vi "DC.vi"(5 "结束冷却":bool, 6 "文本（TSDC）路径：":path=path "C:/Users/Scrooge/Desktop/TSDC.txt", 7 "Ctl Refnum":refnum<vi>, 8 "error in (no error)":errorcluster caption="错误输入（无错误）", 9 "结束温度":dbl, 10 "簇 2":T1, 11 "簇":T2) -> (0 "error out":errorcluster caption="错误输出", 2 "极化电流":dbl, 3 "簇 3":cluster{"当前温度":dbl, "当前电压":bool, "剩余时间":dbl})   [LabVIEW 2017]
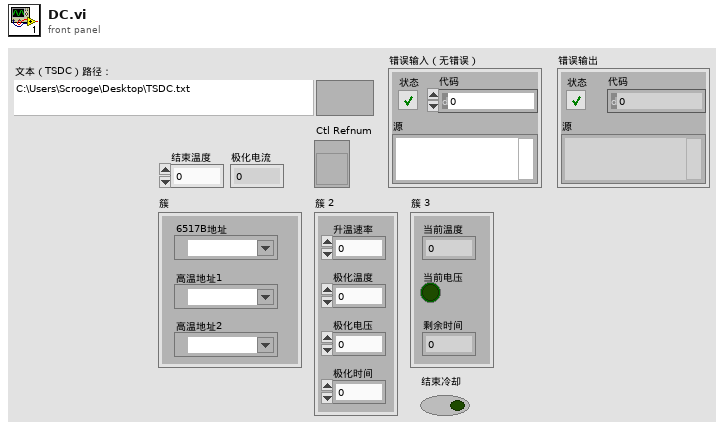
[diagram p1: front panel]
types:
  T1 = cluster{"升温速率":dbl, "极化温度":dbl, "极化电压":dbl, "极化时间":dbl}
  T2 = cluster{"6517B地址":refnum<visa-resource-name>, "高温地址1":refnum<visa-resource-name>, "高温地址2":refnum<visa-resource-name>}
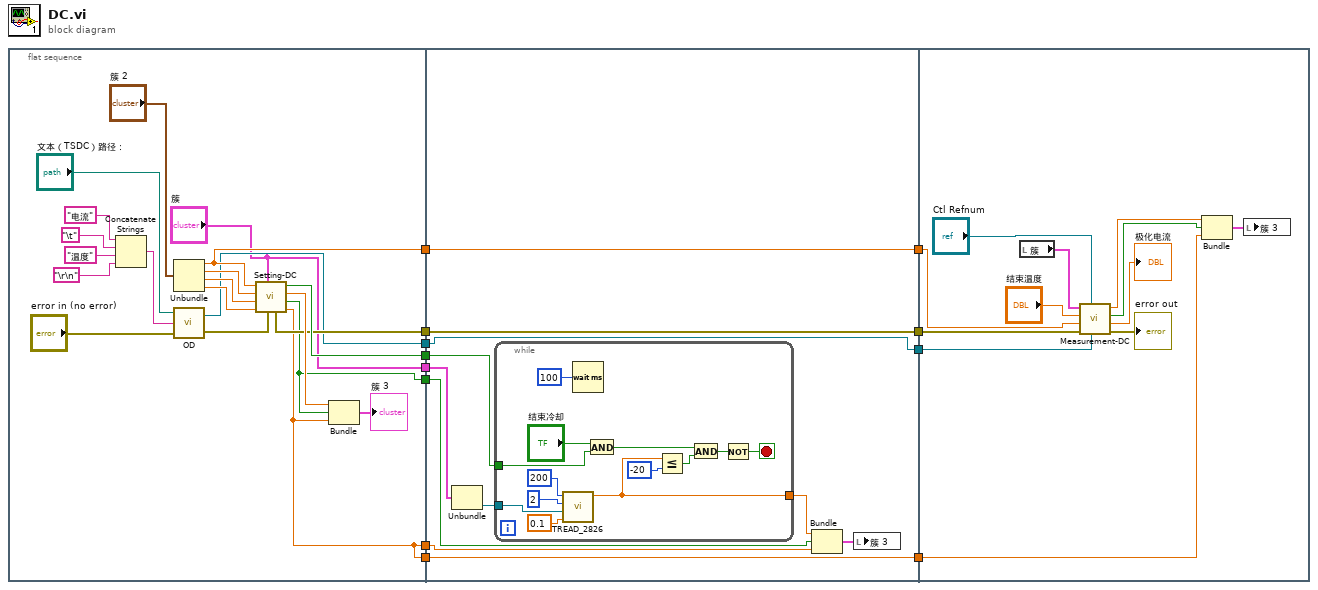
[diagram p0: block diagram]
diagram:
  n1 = flat-sequence {
    tunnel: [w33] -> w12
    tunnel: [w13] -> w10
    tunnel: [w26] -> w8
    tunnel: [w25] -> w6
    tunnel: [w23] -> w4
    tunnel: ["簇"] -> w3
    tunnel: [w14] -> w2
    tunnel: [w13] -> w1
    tunnel: w12 -> [w44]
    tunnel: [w43] -> w11
    tunnel: w10 -> [w43]
    tunnel: [w42] -> w9
    tunnel: w8 -> [w42]
    tunnel: [w41] -> w7
    tunnel: w6 -> [w41]
    tunnel: [w40] -> w5
    tunnel: w4 -> [w40]
    tunnel: w3 -> [w39]
    tunnel: w2 -> [w36]
    tunnel: w1 -> [w35]
    tunnel: w11 -> [w67]
    tunnel: w9 -> [w64]
    tunnel: w7 -> [w63]
    tunnel: w5 -> [w58]
    frame #0 {
      n2 = Concatenate Strings("电流", "\t", "温度" ("字符串"), "\r\n") -> (w20:string)
      n3 = Unbundle("簇 2") -> ("升温速率"=w25:dbl, "极化温度"=w31:dbl, "极化电压"=w30:dbl, "极化时间"=w29:dbl)
      n4 = call "OD.vi"("error in (no error)"="error in (no error)", "字符串"=w20, "路径"="文本（TSDC）路径：") -> ("error out"=w22:errorcluster, "引用句柄输出"=w23:refnum<file>)
      n5 = call "Setting-DC.vi"("error in (no error)"=w22, "簇"="簇", "极化时间"=w29, "极化电压"=w30, "极化温度"=w31, "变温速率"=w25) -> ("剩余时间"=w13:dbl, "当前电压"=w14:bool, "当前温度"=w28:dbl, "极化完毕"=w33:bool, "error out"=w26:errorcluster)  [unwired: 1 in]
      n6 = Bundle("当前温度"=w28, "当前电压"=w14, "剩余时间"=w13) -> (→"簇 3":cluster{"当前温度":dbl, "当前电压":bool, "剩余时间":dbl})  [unwired: 1 in]
    }
    frame #1 {
      n7 = Unbundle(w39) -> ("高温地址2"=w38:refnum<visa-resource-name>)  [unwired: 2 out]
      n8 = while {
        tunnel: w44 -> [w54]
        tunnel: w38 -> [w51]
        tunnel: [w47] -> w37
        stop <- w57 stop-if-true
        n9 = call "TREAD_2826.vi"("Unknown Param 2"=0.1, "VISA resource name"=w51, "Address No."=2, "Unknown Param"=200) -> ("PV"=w47:dbl)  [unwired: 3 out]
        n10 = Wait (ms)(milliseconds to wait=100) -> ()  [unwired: 1 out]
        n11 = And(x="结束冷却", y=w54) -> (x .and. y?=w49:bool)
        n12 = Less Or Equal?(x=w47, y=-20) -> (x <= y?=w45:bool)
        n13 = And(x=w49, y=w45) -> (x .and. y?=w48:bool)
        n14 = Not(x=w48) -> (.not. x?=w57:bool)
      }
      n15 = Bundle("PV"=w37, "当前电压"=w36, "剩余时间"=w35) -> (w34:cluster{"PV":dbl, "当前电压":bool, "剩余时间":dbl})  [unwired: 1 in]
      n16 = local write "簇 3"(w34) -> ()
    }
    frame #2 {
      n17 = local read "簇"() -> (w65:T2)
      n18 = call "Measurement-DC.vi"("引用句柄输出"=w58, "Ctl Refnum"="Ctl Refnum", "error in (no error)"=w64, "升温速率"=w63, "结束温度"="结束温度", "簇"=w65) -> ("error out"=→"error out":errorcluster, "极化电流"=→"极化电流":dbl, "布尔"=w68:bool, "当前温度"=w69:dbl)  [unwired: 2 in]
      n19 = Bundle("当前温度"=w69, "布尔"=w68, "剩余时间"=w67) -> (w66:cluster{"当前温度":dbl, "布尔":bool, "剩余时间":dbl})  [unwired: 1 in]
      n20 = local write "簇 3"(w66) -> ()
    }
  }
